vi "scan current(SubVI).vi"(0 "config in":T1={"initialize"=enum."SR830", "6221"={"6221 Resource"="GPIB0::24::INSTR", "Delta status"=FALSE, "电流"=0.0}, "SR830+6221"={"source"=0, "阻抗"=0.0, "量程入 4"=0, "量程入 3"=0, "量程入 2"=0, "量程入 1"=0, "SR830 2"=FALSE, "SR830 3"=FALSE, "SR830 4"=FALSE, "SR830 1"=FALSE, "VISA 1"="", "VISA 2"="", "VISA 3"="", "VISA 4"="", "Reserve 1"=0, "Reserve 2"=-1, "Reserve 3"=-1, "Reserve 4"=-1, "量程"=enum."量程每次测量会判定"}, "2400"={"2400"=FALSE, "VISA"=""}, "ch"={"ch"=[], "current"=[], "change?"=[], "holding current\nwhen change ch?"=FALSE}, "Instrument"={"335 Resource"="GPIB0::24::INSTR", "Input (0:A)"=0, "Instrument Type"=enum."SVSM", "quantum design"=refnum, "Heater Output (1:1)"=1, "semaphore"=refnum, "TCP master instance"=refnum, "335 Status"=refnum, "M24C Resource"="GPIB0::24::INSTR", "4G supply"="GPIB0::24::INSTR", "Temp Status 24C"=refnum, "Temp"=refnum, "9T信号"=refnum, "limit"={"Field limit"=0.0, "Field rate limit"=0.0, "Temp limit"=0.0, "Temp low limit"=0.0, "Temp rate limit "=0.0}, "4g supply status"=refnum}, "Aborting"=refnum, "数据文件"=refnum, "warning"=refnum} {"Instrument"."Input (0:A)" items=["A", "B"]; "Instrument"."Heater Output (1:1)" items=["1"=1, "2"=2]; "SR830+6221"."Reserve 4" items=["Auto Reserve"=-1, "High Reserve"=0, "Normal"=1, "Low Noise"=2]; "SR830+6221"."Reserve 3" items=["Auto Reserve"=-1, "High Reserve"=0, "Normal"=1, "Low Noise"=2]; "SR830+6221"."Reserve 2" items=["Auto Reserve"=-1, "High Reserve"=0, "Normal"=1, "Low Noise"=2]; "SR830+6221"."Reserve 1" items=["量程每次测量会判定", "量程不变为设定值"]; "SR830+6221"."source" items=["SR830 1", "SR830 2", "SR830 3", "SR830 4"]}, 1 "Current":dbl=300.0, 6 "data":refnum<queue>, 7 "Current 2":dbl=300.0, 9 "steps number":i32) -> (4 "config out":T1={"initialize"=enum."SR830", "6221"={"6221 Resource"="GPIB0::24::INSTR", "Delta status"=FALSE, "电流"=0.0}, "SR830+6221"={"source"=0, "阻抗"=0.0, "量程入 4"=0, "量程入 3"=0, "量程入 2"=0, "量程入 1"=0, "SR830 2"=FALSE, "SR830 3"=FALSE, "SR830 4"=FALSE, "SR830 1"=FALSE, "VISA 1"="", "VISA 2"="", "VISA 3"="", "VISA 4"="", "Reserve 1"=0, "Reserve 2"=-1, "Reserve 3"=-1, "Reserve 4"=-1, "量程"=enum."量程每次测量会判定"}, "2400"={"2400"=FALSE, "VISA"=""}, "ch"={"ch"=[], "current"=[], "change?"=[], "holding current\nwhen change ch?"=FALSE}, "Instrument"={"335 Resource"="GPIB0::24::INSTR", "Input (0:A)"=0, "Instrument Type"=enum."SVSM", "quantum design"=refnum, "Heater Output (1:1)"=1, "semaphore"=refnum, "TCP master instance"=refnum, "335 Status"=refnum, "M24C Resource"="GPIB0::24::INSTR", "4G supply"="GPIB0::24::INSTR", "Temp Status 24C"=refnum, "Temp"=refnum, "9T信号"=refnum, "limit"={"Field limit"=0.0, "Field rate limit"=0.0, "Temp limit"=0.0, "Temp low limit"=0.0, "Temp rate limit "=0.0}, "4g supply status"=refnum}, "Aborting"=refnum, "数据文件"=refnum, "warning"=refnum} {"Instrument"."Input (0:A)" items=["A", "B"]; "Instrument"."Heater Output (1:1)" items=["1"=1, "2"=2]; "SR830+6221"."Reserve 4" items=["Auto Reserve"=-1, "High Reserve"=0, "Normal"=1, "Low Noise"=2]; "SR830+6221"."Reserve 3" items=["Auto Reserve"=-1, "High Reserve"=0, "Normal"=1, "Low Noise"=2]; "SR830+6221"."Reserve 2" items=["Auto Reserve"=-1, "High Reserve"=0, "Normal"=1, "Low Noise"=2]; "SR830+6221"."Reserve 1" items=["量程每次测量会判定", "量程不变为设定值"]; "SR830+6221"."source" items=["SR830 1", "SR830 2", "SR830 3", "SR830 4"]}, 8 "错误输出":errorcluster)   [LabVIEW 2019, in "Scan.lvlib"]
uses:
  Scan.lvlib
  config.ctl
  <vilib>/NI/Modbus Library/API/Master/Modbus Master.lvclass
  initialize.ctl
  Instrument.ctl
  Instrument Type.ctl
  lib/QDInstrument.dll
  335 state.ctl
  limit.ctl
  9T mag field stauts.ctl
  warning.ctl
  SubVI.lvlib
panel:
  out "数组":dbl[](array[numeric])
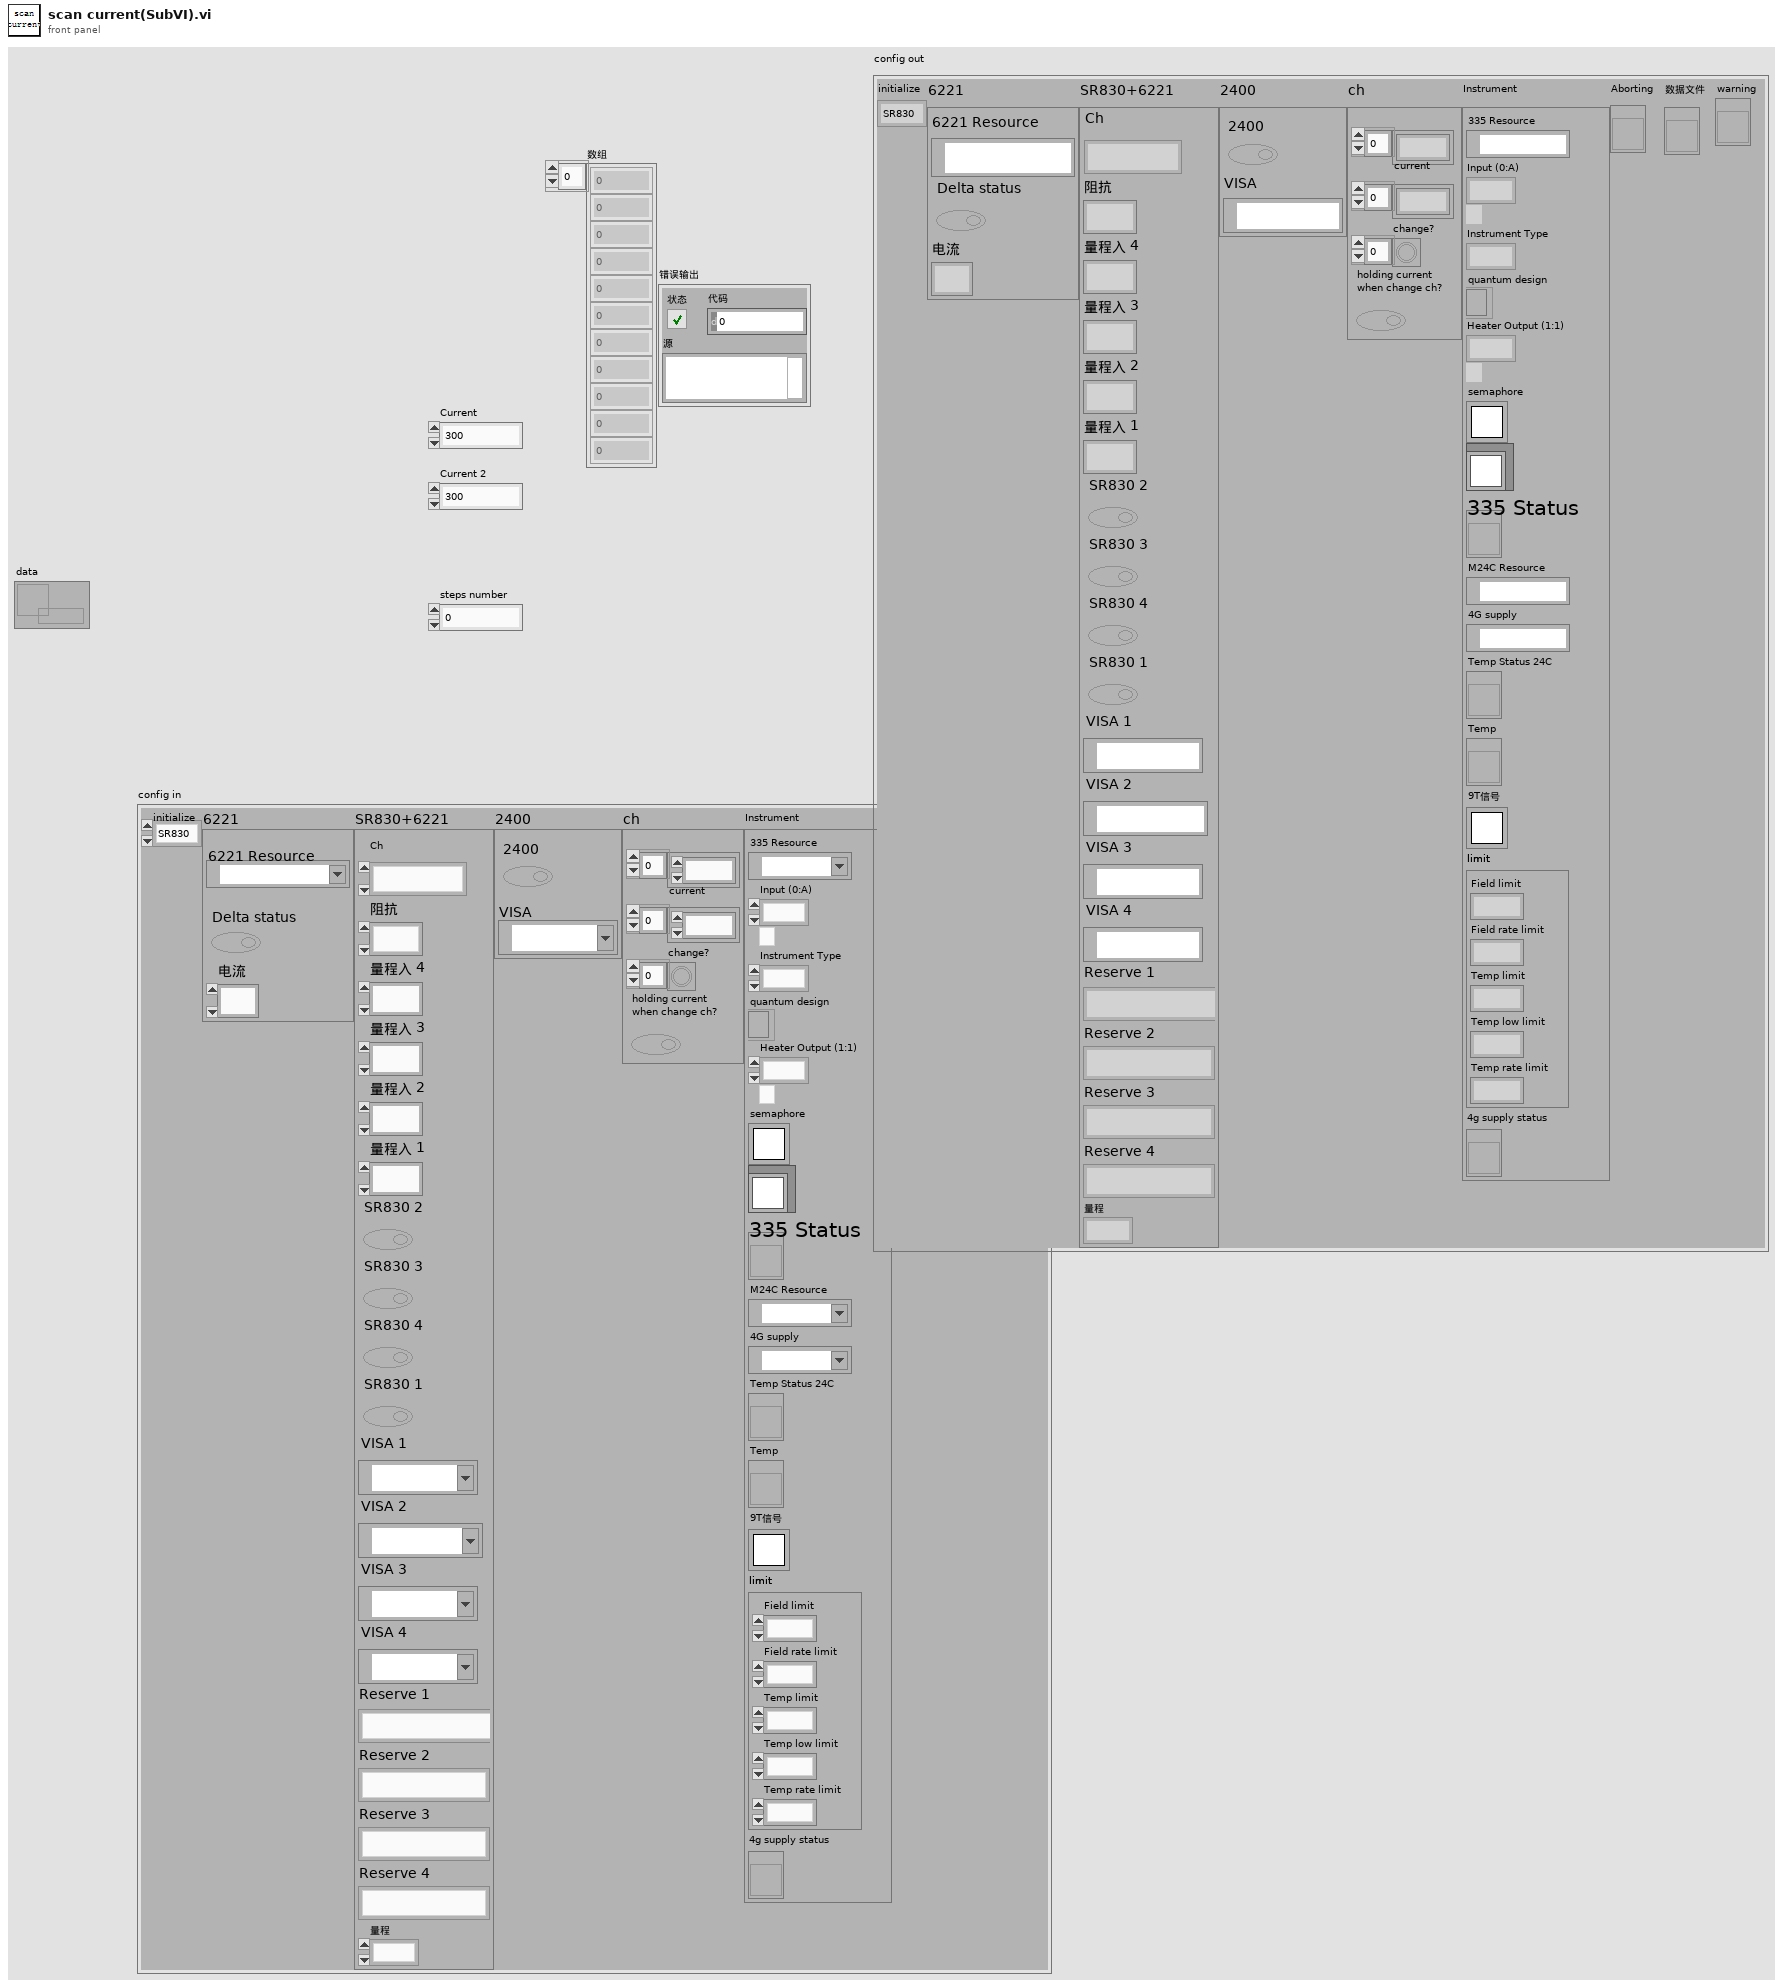
[diagram p1: front panel]
types:
  T1 = typedef "config.ctl" = cluster{"initialize":T2, "6221":cluster{"6221 Resource":refnum<visa-resource-name>, "Delta status":bool, "电流":dbl}, "SR830+6221":cluster{"source":u16, "阻抗":dbl, "量程入 4":i32, "量程入 3":i32, "量程入 2":i32, "量程入 1":i32, "SR830 2":bool, "SR830 3":bool, "SR830 4":bool, "SR830 1":bool, "VISA 1":refnum<visa-resource-name>, "VISA 2":refnum<visa-resource-name>, "VISA 3":refnum<visa-resource-name>, "VISA 4":refnum<visa-resource-name>, "Reserve 1":i16, "Reserve 2":i16, "Reserve 3":i16, "Reserve 4":i16, "量程":enum16{"量程每次测量会判定", "量程不变为设定值"}}, "2400":cluster{"2400":bool, "VISA":refnum<visa-resource-name>}, "ch":cluster{"ch":i32[], "current":dbl[], "change?":bool[], "holding current\nwhen change ch?":bool}, "Instrument":T3, "Aborting":refnum<vi>, "数据文件":refnum<vi>, "warning":refnum<vi>}
  T2 = typedef "initialize.ctl" = enum16{"SR830", "keithley6221-SR830", "Delta", "Delta-tunnelling", "keithley6221-2182-DC"}
  T3 = typedef "Instrument.ctl" = cluster{"335 Resource":refnum<visa-resource-name>, "Input (0:A)":u16, "Instrument Type":T4, "quantum design":refnum<k24>, "Heater Output (1:1)":u16, "semaphore":T5, "TCP master instance":refnum<class "Modbus Master.lvclass">, "335 Status":refnum<vi>, "M24C Resource":refnum<visa-resource-name>, "4G supply":refnum<visa-resource-name>, "Temp Status 24C":refnum<vi>, "Temp":refnum<vi>, "9T信号":T5, "limit":T6, "4g supply status":refnum<vi>}
  T4 = typedef "Instrument Type.ctl" = enum16{"PPMS", "VersaLab", "DynaCool", "SVSM", "PPMS-Rotate", "Lakeshore335", "9T mag"}
  T5 = typedef "Semaphore RefNum" = refnum<k1>
  T6 = typedef "limit.ctl" = cluster{"Field limit":dbl, "Field rate limit":dbl, "Temp limit":dbl, "Temp low limit":dbl, "Temp rate limit ":dbl}
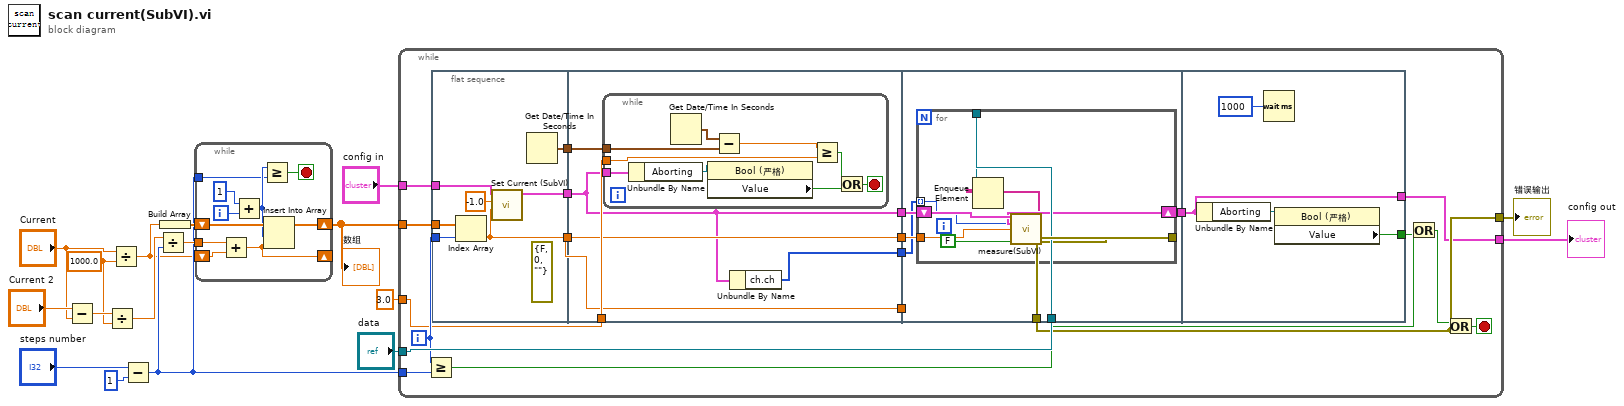
[diagram p0: block diagram]
diagram:
  w6 = 1000.0 ("y")
  n1 = Subtract(x="Current 2", y="Current") -> (x-y=w7:dbl)
  n2 = Divide(x=w7, y=w6) -> (x/y=w5:dbl)
  n3 = Divide(x="Current", y=w6) -> (x/y=w3:dbl)
  n4 = Subtract(x="steps number", y=1) -> (x-y=w10:i32)
  n5 = Divide(x=w5, y=w10) -> (x/y=w17:dbl)
  n6 = Build Array(w3) -> (w16:dbl[])
  n7 = while {
    shift-right: [w27] -> w14
    shift-left: w16 -> [w26]
    tunnel: w17 -> [w21]
    tunnel: w10 -> [w20]
    shift-right: [w19] -> _
    shift-left: w3 -> [w18]
    i -> [w25]
    stop <- w22 stop-if-true
    n8 = Add(x=w21, y=w18) -> (x+y=w19:dbl)
    n9 = Add(x=1, y=w25) -> (x+y=w23:i32)
    n10 = Greater Or Equal?(x=w23, y=w20) -> (x >= y?=w22:bool)
    n11 = Insert Into Array(array=w26, index=w23, new element=w19) -> (w27:dbl[])
  }
  "数组" <- w14
  n12 = while {
    tunnel: w10 -> [w45]
    tunnel: "data" -> [w47]
    tunnel: w14 -> [w43]
    tunnel: [w37] -> w13
    tunnel: 3.0 ("Delay") -> [w40]
    tunnel: "config in" -> [w35]
    tunnel: [w30] -> w1
    i -> [w44]
    stop <- w42 stop-if-true
    n13 = Greater Or Equal?(x=w44, y=w45) -> (x >= y?=w46:bool)
    n14 = flat-sequence {
      tunnel: w44 -> [w53]
      tunnel: w43 -> [w54]
      tunnel: [w52] -> w41
      tunnel: [w51] -> w39
      tunnel: w35 -> [w49]
      tunnel: [w48] -> w34
      tunnel: w41 -> [w59]
      tunnel: w40 -> [w58]
      tunnel: w39 -> [w57]
      tunnel: [w57] -> w38
      tunnel: w34 -> [w56]
      tunnel: [w56] -> w33
      tunnel: [w57] -> w29
      tunnel: [w55] -> w28
      tunnel: w47 -> [w70]
      tunnel: [w74] -> w37
      tunnel: w38 -> [_]
      tunnel: w33 -> [w73]
      tunnel: [w72] -> w32
      tunnel: w29 -> [w71]
      tunnel: w28 -> [w69]
      tunnel: w32 -> [w83]
      tunnel: [w84] -> w31
      tunnel: [w83] -> w30
      frame #0 {
        (unwired) errorcluster {"status"=FALSE, "code"=0, "source"=""} ("error in (no error)")
        n15 = Index Array(array=w54, index=w53) -> (element=w51:dbl)
        n16 = call "Set Current (SubVI).vi"("current(A)"=w51, "freq"=-1.0, "config"=w49) -> ("输出簇"=w48:T1)  [unwired: 8 in]
        n17 = Get Date/Time In Seconds() -> (seconds since 1Jan1904=w52:timestamp)
      }
      frame #1 {
        n18 = while {
          tunnel: w59 -> [w67]
          tunnel: w58 -> [w65]
          tunnel: w56 -> [w62]
          stop <- w63 stop-if-true
          n19 = Unbundle By Name(w62) -> ("Aborting"=w61:refnum<vi>)
          n20 = Get Date/Time In Seconds() -> (seconds since 1Jan1904=w68:timestamp)
          n21 = property class="Bool (严格)"(reference=w61) -> ("Value"=w60:bool)  [unwired: 1 in, 2 out]
          n22 = Subtract(x=w68, y=w67) -> (x-y=w66:dbl)
          n23 = Greater Or Equal?(x=w66, y=w65) -> (x >= y?=w64:bool)
          n24 = Or(x=w64, y=w60) -> (x .or. y?=w63:bool)
        }
        n25 = Unbundle By Name(w56) -> ("ch.ch"=w55:i32[])
      }
      frame #2 {
        n26 = for {
          tunnel: [w82] -> w74
          tunnel: w71 -> [w79]
          shift-right: [w80] -> w72
          shift-left: w73 -> [w81]
          tunnel: w70 -> [w77]
          tunnel: w69 -> [w75] mode=indexing
          n27 = call "measure(SubVI).vi"("config in"=w81, "ch"=w75, "current"=w79, "change?"=FALSE) -> ("data"=w76:string[], "config out"=w80:T1, "error out"=w82:errorcluster)  [unwired: 9 in]
          n28 = Enqueue Element(queue=w77, element=w76) -> ()  [unwired: 2 in, 3 out]
        }
      }
      frame #3 {
        n29 = Unbundle By Name(w83) -> ("Aborting"=w85:refnum<vi>)
        n30 = Wait (ms)(milliseconds to wait=u32 1000 ("等待时间（毫秒）")) -> ()  [unwired: 1 out]
        n31 = property class="Bool (严格)"(reference=w85) -> ("Value"=w84:bool)  [unwired: 1 in, 2 out]
      }
    }
    n32 = Or(x=w46, y=w31) -> (x .or. y?=w36:bool)
    n33 = Or(x=w36, y=w37) -> (x .or. y?=w42:bool)
  }
  "错误输出" <- w13
  "config out" <- w1
